vi "Microscopy.Recognize Digital Trigger.vi"(6 "acq.Trigger Invert":bool, 8 "Data Valid":bool, 11 "TRIG IN":T1) -> (0 "Data Valid Out":bool, 2 "Trig Offset":u8, 3 "RefTrig":bool)   [LabVIEW 2012]
doc: "This VI checks for any rising edge on the digital trigger line. Also, it outputs a trigger offset position in the two parallel samples."
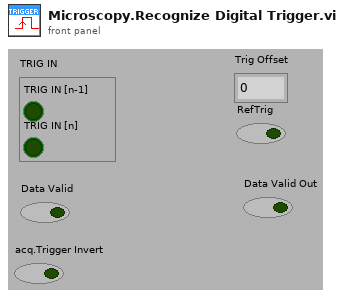
[diagram p1: front panel]
types:
  T1 = cluster{"TRIG IN [n-1]":bool, "TRIG IN [n]":bool}
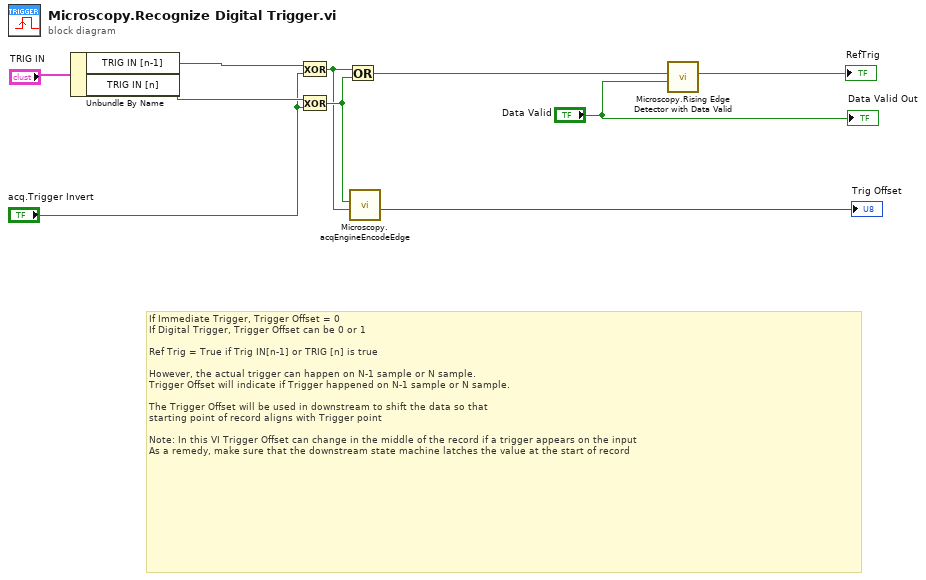
[diagram p0: block diagram]
diagram:
  # "If Immediate Trigger, Trigger Offset = 0\nIf Digital Trigger, Trigger Offset can be 0 or 1\n\nRef Trig = True if Trig IN[n-1] or TRIG [n] is true\n\nHowever, the actual trigger can happen on N-1 sample or N sample.\nTrigger Offset will indicate if Trigger happened on N-1 sample or N sample.\n\nThe Trigger Offset will be used in downstream to shift the data so that\nstarting point of record aligns with Trigger point\n\nNote: In this VI Trigger Offset can change in the middle of the record if a trigger appears on the input\nAs a remedy, make sure that the downstream state machine latches the value at the start of record"
  n1 = Unbundle By Name("TRIG IN") -> ("TRIG IN [n-1]"=w9:bool, "TRIG IN [n]"=w10:bool)
  n2 = Exclusive Or(1:"acq.Trigger Invert", 2:w9) -> (0:w5:bool)
  n3 = Exclusive Or(1:"acq.Trigger Invert", 2:w10) -> (0:w6:bool)
  n4 = Or(x=w5, y=w6) -> (x .or. y?=w7:bool)
  n5 = call "Microscopy.acqEngineEncodeEdge.vi"("Early RefTrig?"=w5, "Later RefTrig?"=w6) -> ("Trig Offset"=→"Trig Offset":u8)  [unwired: 8 in, 1 out]
  n6 = call "Microscopy.Rising Edge Detector with Data Valid.vi"("Data Valid"="Data Valid", "signal"=w7) -> ("edge detected"=→"RefTrig":bool)  [unwired: 9 in]
  "Data Valid Out" <- "Data Valid"
